vi "ChooseDualXDCRSettings.vi"(0 "Digitizer Settings in":T22={"Digitizer delay (us) "=0.0, "rf points per line"=0, "lines per plane"=0, "Samp Rate (Hz)"=0.0, "Additional dig delay (us)"=0.0, "Voltage Scale"=0.0, "Pre-Looks"=0, "Offset delay (us)"=0.0, "bits A/D"=0, "Avg Num"=0, "DigTimeOut"=0.0, "Rel Dig Delay"=0.0, "Dig Ch"=0, "LeCroyCluster"={"LeCroy Channels"=[], "LC read pt offset"=0.0, "Sweep Avg"=FALSE}, "Main Digitizer"=enum."Acqiris Digitizer", "Dig Config"=enum."Single channel", "Digitizer ID Cluster"={"Acqiris/Alazar/SP ID"=[], "NI Instr Handles"=[], "LeCroy VISA"="", "GaGe Handle"={"Handle"=0, "Sample size"=0, "Resolution"=0, "Offset"=0, "Channels"=0, "Boards"=0}, "ATS Ref"="ATS9350", "Acqiris Address"=["PCI::INSTR0"], "ADQRef"=refnum, "adq_cu_ptr"=refnum}, "Trigger Settings"={"Trig Source"=0, "Trig Coupling"=0, "Trig Slope"=0, "Level (mV)"=0.0}, "Bulk Acq"=FALSE, "Bulk Start Indexes"=[], "Data Ref RF"=refnum, "NI ID/Channel"=[], "Total Dig CH"=1, "Xtra Ann Trig delay (us)"=10.0, "Fix Z Delay?"=FALSE, "One Way Transmission?"=FALSE, "Data Ref Log"=refnum} {"Trigger Settings"."Trig Slope" items=["Positive", "Negative"]; "Trigger Settings"."Level (mV)" format="%.2f"; "Trigger Settings"."Trig Coupling" items=["DC 1 MOhm", "AC 1 MOhm", "DC 50 Ohm", "AC 50 Ohm"]; "Trigger Settings"."Trig Source" items=["Chan 1", "External"]; "Rel Dig Delay" format="%.2f"; "DigTimeOut" format="%.2f"; "Avg Num" min=1; "Offset delay (us)" format="%.2f"; "Additional dig delay (us)" format="%.2f"; "Digitizer delay (us)" format="%.2f"}, 1 "Switch T/R":u32=1, 2 "Set All UTEX?":bool=TRUE, 3 "Pulser":T1, 5 "Motion Settings in":T26={"No Motion?"=FALSE, "Motion System"=enum."MM3000", "Motion Bd ID"=0, "Motion Profile"="SMAC1", "# Axis"=0, "Reverse Z axis?"=FALSE, "SMAC Axis"=0, "scan pair"=enum."y-(x) scan", "RT fps"=0.0, "Steps per mm"=[], "Motor Parameters"={"velocity ct/s"=[], "accel ct/s^2"=[]}, "One Way Scan"=FALSE, "Reverse One Way Scan"=FALSE, "Global Position (mm)"=[], "Plane"=0, "Distance between\nscan lines (um)"=0.0, "Distance between\nscan planes (um)"=0.0, "number of scan planes"=0, "Total steps in line"=0, "Xtra plane\ndistance  (um)"=0, "Xtra planes "=0, "Add Axis"=FALSE, "overshoot cts"=0, "BKPT Shift"=0, "Scan Start Time (ms)"=0, "ESP VISA"="", "3rd Axis"=1, "GL Ref Out"=refnum, "Galil Address"=""} {"3rd Axis" items=["x", "y", "z", "w"]; "Xtra planes" min=1; "Xtra plane\ndistance  (um)" min=0; "Distance between\nscan planes (um)" format="%.2f"; "Distance between\nscan lines (um)" format="%.2f"; "SMAC Axis" items=["None"=0, "Axis 1"=1, "Axis 2"=2, "Axis 3"=3, "Axis 4"=4, "Axis 5"=5, "Axis 6"=6, "Axis 7"=7, "Axis 8"=8, "Vector Space 1"=17, "Vector Space 2"=18, "Vector Space 3"=19, "Vector Space 4"=20]; "Motion Bd ID" min=1 max=32 step=1}, 7 "Dual XDCR Settings":T2 {"XDCR Settings"."UT340 Controls"."Low Pass Filter (MHz)" min=-6 max=60 step=1; "XDCR Settings"."UT340 Controls"."High Pass Filter (MHz)" min=1 max=20 step=1; "XDCR Settings"."UT340 Controls"."Rep Rate (Hz)" min=20 step=1; "XDCR Settings"."UT340 Controls"."Pulse Width (ns)" min=100.0 max=250.0 step=2.0; "XDCR Settings"."UT340 Controls"."Voltage" min=100 max=250 step=2; "XDCR Settings"."UT340 Controls"."PC Gain (dB)" min=2 max=72; "XDCR Settings"."UT340 Controls"."PE Gain (dB)" min=-6 max=60 step=1; "XDCR Settings"."JSR Complete"."JSR Trigger Settings"."PRF (Hz)" items=["100 Hz"=0.1, "200 Hz"=0.2, "400 Hz"=0.4, "600 Hz"=0.6, "800 Hz"=0.8, "1000 Hz"=1.0, "1250 Hz"=1.25, "1500 Hz"=1.5, "1750 Hz"=1.75, "2000 Hz"=2.0, "2500 Hz"=2.5, "3000 Hz"=3.0, "3500 Hz"=3.5, "4000 Hz"=4.0, "4500 Hz"=4.5, "5000 Hz"=5.0]; "XDCR Settings"."JSR Complete"."JSR Trigger Settings"."Trigger Source" items=["Internal", "External"]; "XDCR Settings"."JSR Complete"."JSR Trigger Settings"."External Trigger Limit" items=["No Limit", "5 kHz"]; "XDCR Settings"."JSR Complete"."JSR Receive Settings"."Gain (dB)" min=-13 max=66 step=1; "XDCR Settings"."JSR Complete"."JSR Receive Settings"."Low Pass Filter" items=["5 MHz"=5, "10 MHz"=10, "15 MHz"=15, "22.5 MHz"=22, "35 MHz"=35, "50 MHz"=50]; "XDCR Settings"."JSR Complete"."JSR Receive Settings"."High Pass Filter" items=["DC"=0, "1 MHz"=1000, "2.5 MHz"=2500, "5 MHz"=5000, "7.5 MHz"=7500, "12.5 MHz"=12500]; "XDCR Settings"."JSR Complete"."JSR Receive Settings"."Receiver Mode" items=["Echo", "Through"]; "XDCR Settings"."JSR Complete"."JSR Pulse Settings"."Pulser Voltage (V)" items=["100"=100, "125"=125, "150"=150, "175"=175, "200"=200, "225"=225, "250"=250, "275"=275, "300"=300, "325"=325, "350"=350, "375"=375, "400"=400, "425"=425, "450"=450, "475"=475]; "XDCR Settings"."JSR Complete"."JSR Pulse Settings"."Pulser Impedance" items=["High z", "Low z"]; "XDCR Settings"."JSR Complete"."JSR Pulse Settings"."Pulse Energy Level" items=["0 (Minimum)", "1", "2", "3 (Maximum)"]; "XDCR Settings"."JSR Complete"."JSR Pulse Settings"."Damping" items=["331 Ohms"=331, "198 Ohms"=198, "142 Ohms"=142, "110 Ohms"=110, "92 Ohms"=92, "77 Ohms"=77, "67 Ohms"=67, "59 Ohms"=59, "52 Ohms"=52, "47 Ohms"=47, "43 Ohms"=43, "39 Ohms"=39, "37 Ohms"=37, "34 Ohms"=34, "32 Ohms"=32, "30 Ohms"=30]; "XDCR Settings"."Panametrics Settings"."FINE ATTENUATION" items=["00.0", "00.5", "01.0", "01.5", "02.0", "02.5", "03.0", "03.5", "04.0", "04.5", "05.0", "05.5", "06.0", "06.5", "07.0", "07.5", "08.0", "08.5", "09.0", "09.5", "10.0", "10.5", "11.0", "11.5", "12.0", "12.5", "13.0", "13.5", "14.0", "14.5", "15.0", "15.5"]; "XDCR Settings"."Panametrics Settings"."COARSE ATTENUATION" items=["00.0", "10.0", "20.0", "30.0", "40.0", "50.0"]; "XDCR Settings"."Panametrics Settings"."GAIN (db)" items=["26.0", "40.0", "54.0"]; "XDCR Settings"."Panametrics Settings"."PRF (KHz)" items=["XREMT", "EXBNC", "0.200", "0.500", "1.000", "2.000", "5.000", "10.00", "20.00"]; "XDCR Settings"."Panametrics Settings"."MODE" items=["P/ E", "THRU", "RPP", "EXT_PLSR"]; "XDCR Settings"."Panametrics Settings"."LP FILT (MHz)" items=["20", "50", "100", "200"]; "XDCR Settings"."Panametrics Settings"."HP FILT (KHz)" items=["1", "1000", "3000", "10000"]; "XDCR Settings"."Panametrics Settings"."DAMPING (Ohm)" items=["7", "10", "16", "20", "26", "30", "40", "50"]; "XDCR Settings"."Panametrics Settings"."ENERGY (uJ)" items=["1", "2", "4", "8", "16", "32"]; "XDCR Settings"."Daxsonics Settings"."Freq (MHz)" items=["4"=4, "5"=5, "6"=6, "8"=8, "10"=10, "12"=12, "14"=14, "15"=15, "16"=16, "17"=17, "18"=18, "20"=20, "25"=25, "30"=30, "35"=35, "40"=40, "45"=45, "50"=50]; "XDCR Settings"."Daxsonics Settings"."Voltage (V)" items=["0"=0, "5"=5, "10"=10, "15"=15, "20"=20, "25"=25, "30"=30, "35"=35, "40"=40, "45"=45, "50"=50, "55"=55, "60"=60, "65"=65, "70"=70, "75"=75, "80"=80, "85"=85, "90"=90, "95"=95, "100"=100, "110"=110, "120"=120, "130"=130, "140"=140, "150"=150, "160"=160, "170"=170, "180"=180, "190"=190]; "XDCR Settings"."Daxsonics Settings"."Gain (dB)" items=["22"=22, "25"=25, "28"=28, "31"=31, "34"=34, "37"=37, "40"=40, "43"=43, "46"=46, "49"=49, "52"=52, "55"=55, "58"=58, "61"=61, "64"=64, "67"=67]; "XDCR Settings"."Digitizer Settings"."Additional dig delay (ms)" format="%.2f"; "XDCR Settings"."Digitizer Settings"."Time scale per Div" items=["100 ns"=0.1, "200 ns"=0.2, "500 ns"=0.5, "1 micros"=1.0, "2 micros"=2.0, "5 micros"=5.0, "10 micros"=10.0, "20 micros"=20.0, "50 micros"=50.0, "100 micros"=100.0, "200 micros"=200.0, "500 micros"=500.0, "1 ms"=1000.0, "2 ms"=2000.0, "5 ms"=5000.0, "10 ms"=10000.0, "20 ms"=20000.0, "50 ms"=50000.0, "100 ms"=100000.0, "200 ms"=200000.0]; "XDCR Settings"."Digitizer Settings"."RF data Sampling"."rf points per line" min=1; "XDCR Settings"."Digitizer Settings"."RF data Sampling"."Ref Delay (ms)" format="%.2f"}, 8 "Setup Time\nParameters (F)":bool, 9 "Allow USB R/Ws?":bool=TRUE, 10 "JSR Simple":refnum<vi>, 11 "JSR Complete":refnum<vi>, 12 "Time scale per Div Ref":refnum<vi>, 13 "RF data Sampling Ref":refnum<vi>, 14 "Filter Parameters Ref":refnum<vi>, 15 "Daxsonics Settings Ref":refnum<vi>, 16 "Panametrics Simple Ref":refnum<vi>, 17 "Panametrics Settings Ref":refnum<vi>, 18 "UT340 Simple Ref":refnum<vi>, 19 "UT340 Ref":refnum<vi>) -> (20 "Digitizer Settings":T22={"Digitizer delay (us) "=0.0, "rf points per line"=0, "lines per plane"=0, "Samp Rate (Hz)"=0.0, "Additional dig delay (us)"=0.0, "Voltage Scale"=0.0, "Pre-Looks"=0, "Offset delay (us)"=0.0, "bits A/D"=0, "Avg Num"=0, "DigTimeOut"=0.0, "Rel Dig Delay"=0.0, "Dig Ch"=0, "LeCroyCluster"={"LeCroy Channels"=[], "LC read pt offset"=0.0, "Sweep Avg"=FALSE}, "Main Digitizer"=enum."Acqiris Digitizer", "Dig Config"=enum."Single channel", "Digitizer ID Cluster"={"Acqiris/Alazar/SP ID"=[], "NI Instr Handles"=[], "LeCroy VISA"="", "GaGe Handle"={"Handle"=0, "Sample size"=0, "Resolution"=0, "Offset"=0, "Channels"=0, "Boards"=0}, "ATS Ref"="ATS9350", "Acqiris Address"=["PCI::INSTR0"], "ADQRef"=refnum, "adq_cu_ptr"=refnum}, "Trigger Settings"={"Trig Source"=0, "Trig Coupling"=0, "Trig Slope"=0, "Level (mV)"=0.0}, "Bulk Acq"=FALSE, "Bulk Start Indexes"=[], "Data Ref RF"=refnum, "NI ID/Channel"=[], "Total Dig CH"=1, "Xtra Ann Trig delay (us)"=10.0, "Fix Z Delay?"=FALSE, "One Way Transmission?"=FALSE, "Data Ref Log"=refnum} {"Trigger Settings"."Trig Slope" items=["Positive", "Negative"]; "Trigger Settings"."Level (mV)" format="%.2f"; "Trigger Settings"."Trig Coupling" items=["DC 1 MOhm", "AC 1 MOhm", "DC 50 Ohm", "AC 50 Ohm"]; "Trigger Settings"."Trig Source" items=["Chan 1", "External"]; "Rel Dig Delay" format="%.2f"; "DigTimeOut" format="%.2f"; "Avg Num" min=1; "Offset delay (us)" format="%.2f"; "Additional dig delay (us)" format="%.2f"; "Digitizer delay (us)" format="%.2f"}, 21 "Change Polarity":i32, 25 "Motion Settings":T26={"No Motion?"=FALSE, "Motion System"=enum."MM3000", "Motion Bd ID"=0, "Motion Profile"="SMAC1", "# Axis"=0, "Reverse Z axis?"=FALSE, "SMAC Axis"=0, "scan pair"=enum."y-(x) scan", "RT fps"=0.0, "Steps per mm"=[], "Motor Parameters"={"velocity ct/s"=[], "accel ct/s^2"=[]}, "One Way Scan"=FALSE, "Reverse One Way Scan"=FALSE, "Global Position (mm)"=[], "Plane"=0, "Distance between\nscan lines (um)"=0.0, "Distance between\nscan planes (um)"=0.0, "number of scan planes"=0, "Total steps in line"=0, "Xtra plane\ndistance  (um)"=0, "Xtra planes "=0, "Add Axis"=FALSE, "overshoot cts"=0, "BKPT Shift"=0, "Scan Start Time (ms)"=0, "ESP VISA"="", "3rd Axis"=1, "GL Ref Out"=refnum, "Galil Address"=""} {"3rd Axis" items=["x", "y", "z", "w"]; "Xtra planes" min=1; "Xtra plane\ndistance  (um)" min=0; "Distance between\nscan planes (um)" format="%.2f"; "Distance between\nscan lines (um)" format="%.2f"; "SMAC Axis" items=["None"=0, "Axis 1"=1, "Axis 2"=2, "Axis 3"=3, "Axis 4"=4, "Axis 5"=5, "Axis 6"=6, "Axis 7"=7, "Axis 8"=8, "Vector Space 1"=17, "Vector Space 2"=18, "Vector Space 3"=19, "Vector Space 4"=20]; "Motion Bd ID" min=1 max=32 step=1})   [LabVIEW 2022 SP3]
uses:
  Motion Controllers/NI_controller/-NI_MotionRoutines/MotionParameters.ctl
  Motion Controllers/NI_controller/-NI_MotionRoutines/MotionSys.ctl
  Motion Controllers/-MotionRoutines/ScanAxis.ctl
  Motion Controllers/-MotionRoutines/3rdAxis.ctl
  Digitizers/-DigitizerRoutines/DigitizerSettings.ctl
  Digitizers/-DigitizerRoutines/Digitizer.ctl
  Digitizers/-DigitizerRoutines/DigConfig.ctl
  Digitizers/-DigitizerRoutines/DigitizerID.ctl
  C:/Windows/System32/ADQAPI_dotNet_helper.dll
  Windows/System32/ADQAPI_dotNet_helper.dll
  Dual XDCR Complete Settings.ctl
  XDCRSettings.ctl
  Pulsers/Daxsonics/-DaxSubroutines/Dax_Control_Cluster.ctl
  Pulsers/Panametrics/Pana5900.ctl
  Pulsers/JSR/Controls/JSR Complete.ctl
  Pulsers/JSR/Controls/JSR Pulse.ctl
  Pulsers/JSR/Controls/Damping.ctl
  Pulsers/JSR/Controls/Energy.ctl
  Pulsers/JSR/Controls/Z.ctl
  Pulsers/JSR/Controls/Volt.ctl
  Pulsers/JSR/Controls/JSR Recieve.ctl
  Pulsers/JSR/Controls/Mode.ctl
  Pulsers/JSR/Controls/HPF.ctl
  Pulsers/JSR/Controls/LPF.ctl
  Pulsers/JSR/Controls/Gain.ctl
  Pulsers/JSR/Controls/JSR Trigger.ctl
  Pulsers/JSR/Controls/Trig Limit.ctl
  Pulsers/JSR/Controls/Trig Source.ctl
  Pulsers/JSR/Controls/PRF.ctl
  Pulsers/UTEX/Controls/UTEX Controls.ctl
  Pulsers/pulser.ctl
  Pulsers/JSR/Controls/JSR Simple.ctl
  Pulsers/UTEX/Controls/UTEX Controls Simple.ctl
  Pulsers/PulserGlobals.vi
panel:
  # "1-D and 2-D B scan settings"
  # "1-D and 2-D B scan settings"
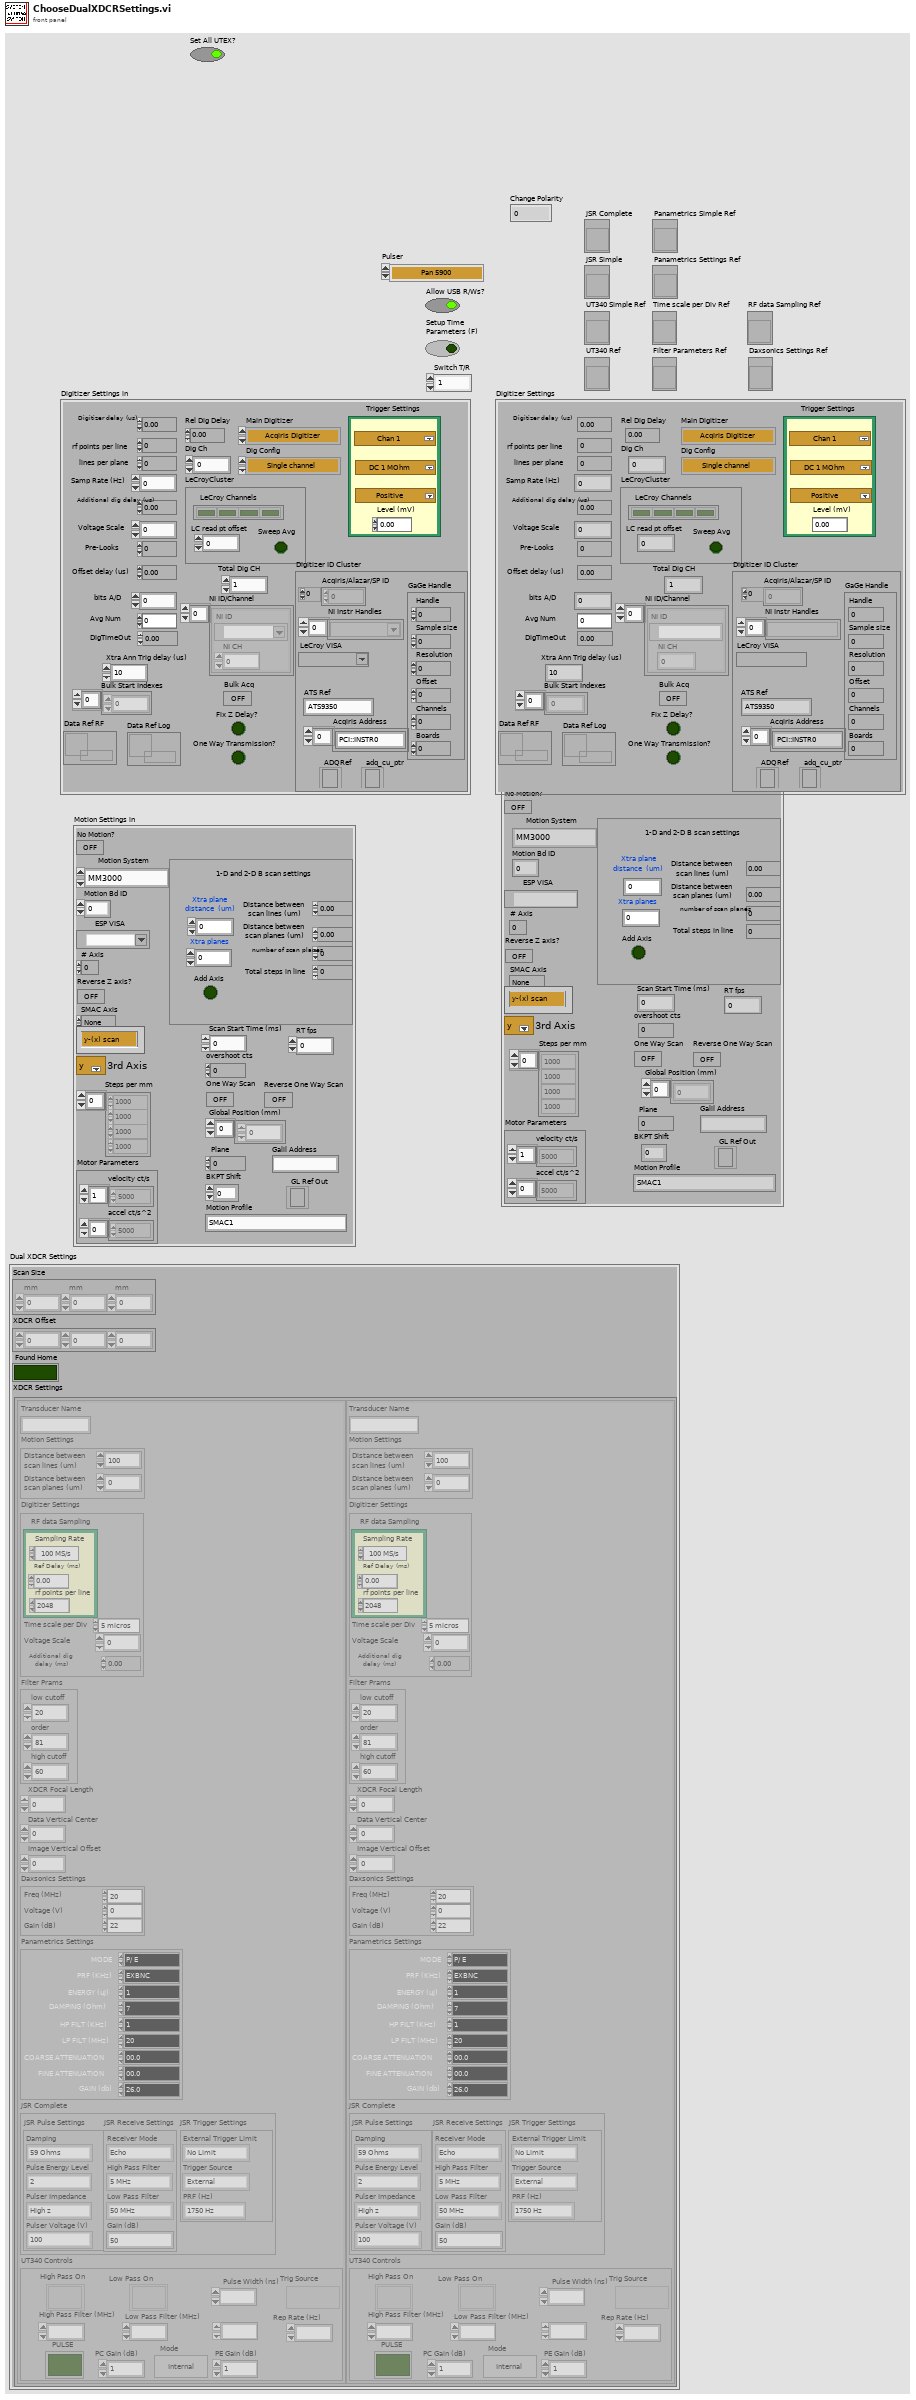
[diagram p1: front panel]
types:
  T1 = typedef "pulser.ctl" = enum16{"Pan 5900", "Daxsonics", "Agilent 33xxx", "UTEX", "JSR", "WMC Mono-Cycle", "No Pulser", "NYU AVTECH", "Tabor W1281A", "Pan 5800", "Unlisted", "Tabor WX2182B"}
  T2 = typedef "Dual XDCR Complete Settings.ctl" = cluster{"Scan Size":dbl[], "XDCR Offset":dbl[], "Found Home":bool, "XDCR Settings":T3[]}
  T3 = typedef "XDCRSettings.ctl" = cluster{"Transducer Name":string, "Motion Settings":cluster{"Distance between\nscan lines (um)":sgl, "Distance between\nscan planes (um)":sgl}, "Digitizer Settings":cluster{"RF data Sampling":cluster{"Sampling Rate":dbl, "Ref Delay (ms)":dbl, "rf points per line":i32}, "Time scale per Div":dbl, "Voltage Scale":dbl, "Additional dig delay (ms)":dbl}, "Filter Prams":cluster{"low cutoff":i32, "order":i32, "high cutoff":i32}, "XDCR Focal Length":dbl, "Data Vertical Center":dbl, "Image Vertical Offset":dbl, "Daxsonics Settings":T4, "Panametrics Settings":T5, "JSR Complete":T6, "UT340 Controls":T21}
  T4 = typedef "Dax_Control_Cluster.ctl" = cluster{"Freq (MHz) ":u16, "Voltage (V)":u16, "Gain (dB)":u16}
  T5 = typedef "Pana5900.ctl" = cluster{"ENERGY (uJ)":u16, "DAMPING (Ohm)":u16, "HP FILT (KHz) ":u16, "LP FILT (MHz)":u16, "MODE":u16, "PRF (KHz)":u16, "GAIN (db)":u16, "COARSE ATTENUATION":u16, "FINE ATTENUATION":u16}
  T6 = typedef "JSR Complete.ctl" = cluster{"JSR Pulse Settings":T7, "JSR Receive Settings":T12, "JSR Trigger Settings":T17}
  T7 = typedef "JSR Pulse.ctl" = cluster{"Damping":T8, "Pulse Energy Level":T9, "Pulser Impedance":T10, "Pulser Voltage (V)":T11}
  T8 = typedef "Damping.ctl" = i16
  T9 = typedef "Energy.ctl" = u16
  T10 = typedef "Z.ctl" = u16
  T11 = typedef "Volt.ctl" = i16
  T12 = typedef "JSR Recieve.ctl" = cluster{"Receiver Mode":T13, "High Pass Filter":T14, "Low Pass Filter":T15, "Gain (dB)":T16}
  T13 = typedef "Mode.ctl" = i8
  T14 = typedef "HPF.ctl" = u16
  T15 = typedef "LPF.ctl" = u16
  T16 = typedef "Gain.ctl" = i8
  T17 = typedef "JSR Trigger.ctl" = cluster{"External Trigger Limit":T18, "Trigger Source":T19, "PRF (Hz)":T20}
  T18 = typedef "Trig Limit.ctl" = i8
  T19 = typedef "Trig Source.ctl" = i8
  T20 = typedef "PRF.ctl" = dbl
  T21 = typedef "UTEX Controls.ctl" = cluster{"High Pass On":bool, "High Pass Filter (MHz)":i16, "Low Pass On":bool, "Low Pass Filter (MHz)":i16, "PE Gain (dB)":i16, "Voltage":i16, "Pulse Width (ns)":dbl, "Mode":bool, "PC Gain (dB)":i16, "Trig Source":bool, "Rep Rate (Hz)":i16, "PULSE":bool}
  T22 = typedef "DigitizerSettings.ctl" = cluster{"Digitizer delay (us) ":dbl, "rf points per line":i32, "lines per plane":i32, "Samp Rate (Hz)":dbl, "Additional dig delay (us)":dbl, "Voltage Scale":dbl, "Pre-Looks":i32, "Offset delay (us)":dbl, "bits A/D":i8, "Avg Num":i32, "DigTimeOut":sgl, "Rel Dig Delay":sgl, "Dig Ch":i32, "LeCroyCluster":cluster{"LeCroy Channels":bool[], "LC read pt offset":dbl, "Sweep Avg":bool}, "Main Digitizer":T23, "Dig Config":T24, "Digitizer ID Cluster":T25, "Trigger Settings":cluster{"Trig Source":u16, "Trig Coupling":u16, "Trig Slope":u16, "Level (mV)":dbl}, "Bulk Acq":bool, "Bulk Start Indexes":i32[], "Data Ref RF":refnum<data-value>, "NI ID/Channel":cluster{"NI ID":refnum<k15>, "NI CH":i32}[], "Total Dig CH":i32, "Xtra Ann Trig delay (us)":dbl, "Fix Z Delay?":bool, "One Way Transmission?":bool, "Data Ref Log":refnum<data-value>}
  T23 = typedef "Digitizer.ctl" = enum16{"Acqiris Digitizer", "NI Digitizer", "LeCroy", "GaGe", "AlazarTech", "No Digitizer", "Teledyne"}
  T24 = typedef "DigConfig.ctl" = enum16{"Single channel", "2 Chans w/ 2 Acqiris", "2 Chans w/ 1 Acqiris", "5-CH Pulser New", "5-CH pulser w/ ann array", "5-pass style ann array", "Empty"}
  T25 = typedef "DigitizerID.ctl" = cluster{"Acqiris/Alazar/SP ID":u32[], "NI Instr Handles":refnum<k15>[], "LeCroy VISA":refnum<visa-resource-name>, "GaGe Handle":cluster{"Handle":u32, "Sample size":u32, "Resolution":i32, "Offset":i32, "Channels":u32, "Boards":u32}, "ATS Ref":string, "Acqiris Address":string[], "ADQRef":refnum<k24>, "adq_cu_ptr":refnum<k24>}
  T26 = typedef "MotionParameters.ctl" = cluster{"No Motion?":bool, "Motion System":T27, "Motion Bd ID":u8, "Motion Profile":string, "# Axis":i8, "Reverse Z axis?":bool, "SMAC Axis":u16, "scan pair":T28, "RT fps":sgl, "Steps per mm":i32[], "Motor Parameters":cluster{"velocity ct/s":dbl[], "accel ct/s^2":dbl[]}, "One Way Scan":bool, "Reverse One Way Scan":bool, "Global Position (mm)":dbl[], "Plane":i32, "Distance between\nscan lines (um)":sgl, "Distance between\nscan planes (um)":sgl, "number of scan planes":i32, "Total steps in line":i32, "Xtra plane\ndistance  (um)":i32, "Xtra planes ":i32, "Add Axis":bool, "overshoot cts":i32, "BKPT Shift":i32, "Scan Start Time (ms)":u32, "ESP VISA":refnum<visa-resource-name>, "3rd Axis":T29, "GL Ref Out":refnum<k7>, "Galil Address":string}
  T27 = typedef "MotionSys.ctl" = enum16{"MM3000", "NI 735x", "Newport ESP", "No Motion Card", "Galil"}
  T28 = typedef "ScanAxis.ctl" = enum16{"y-(x) scan", "x-(y) scan", "z-(x) scan", "z-(y) scan", "y-(z) scan", "x-(z) scan", "w-(x) scan", "w-(y) scan", "w-(z) scan", "x-(w) scan", "y-(w) scan", "z-(w) scan"}
  T29 = typedef "3rdAxis.ctl" = u16
  T30 = cluster{"ENERGY (uJ)":u16, "COARSE ATTENUATION":u16, "FINE ATTENUATION":u16}
  T31 = cluster{"High Pass On":bool, "High Pass Filter (MHz)":bool, "Low Pass On":bool, "Low Pass Filter (MHz)":bool, "PE Gain (dB)":bool, "Voltage":bool, "Pulse Width (ns)":bool, "Mode":bool, "PC Gain (dB)":bool, "Trig Source":bool, "Rep Rate (Hz)":bool, "PULSE":bool}
  T32 = cluster{"RF data Sampling":cluster{"Sampling Rate":dbl, "Ref Delay (ms)":dbl, "rf points per line":i32}, "Time scale per Div":dbl, "Voltage Scale":dbl, "Additional dig delay (ms)":dbl}
  T33 = cluster{"Distance between\nscan lines (um)":sgl, "Distance between\nscan planes (um)":sgl}
  T34 = cluster{"low cutoff":i32, "order":i32, "high cutoff":i32}
  T35 = typedef "JSR Simple.ctl" = cluster{"Pulse Energy Level":T9, "Gain (dB)":T16, "Pulser Voltage (V)":T11}
  T36 = typedef "UTEX Controls Simple.ctl" = cluster{"PE Gain (dB)":i16, "Voltage":i16}
  T37 = cluster{"Sampling Rate":dbl, "Ref Delay (ms)":dbl, "rf points per line":i32}
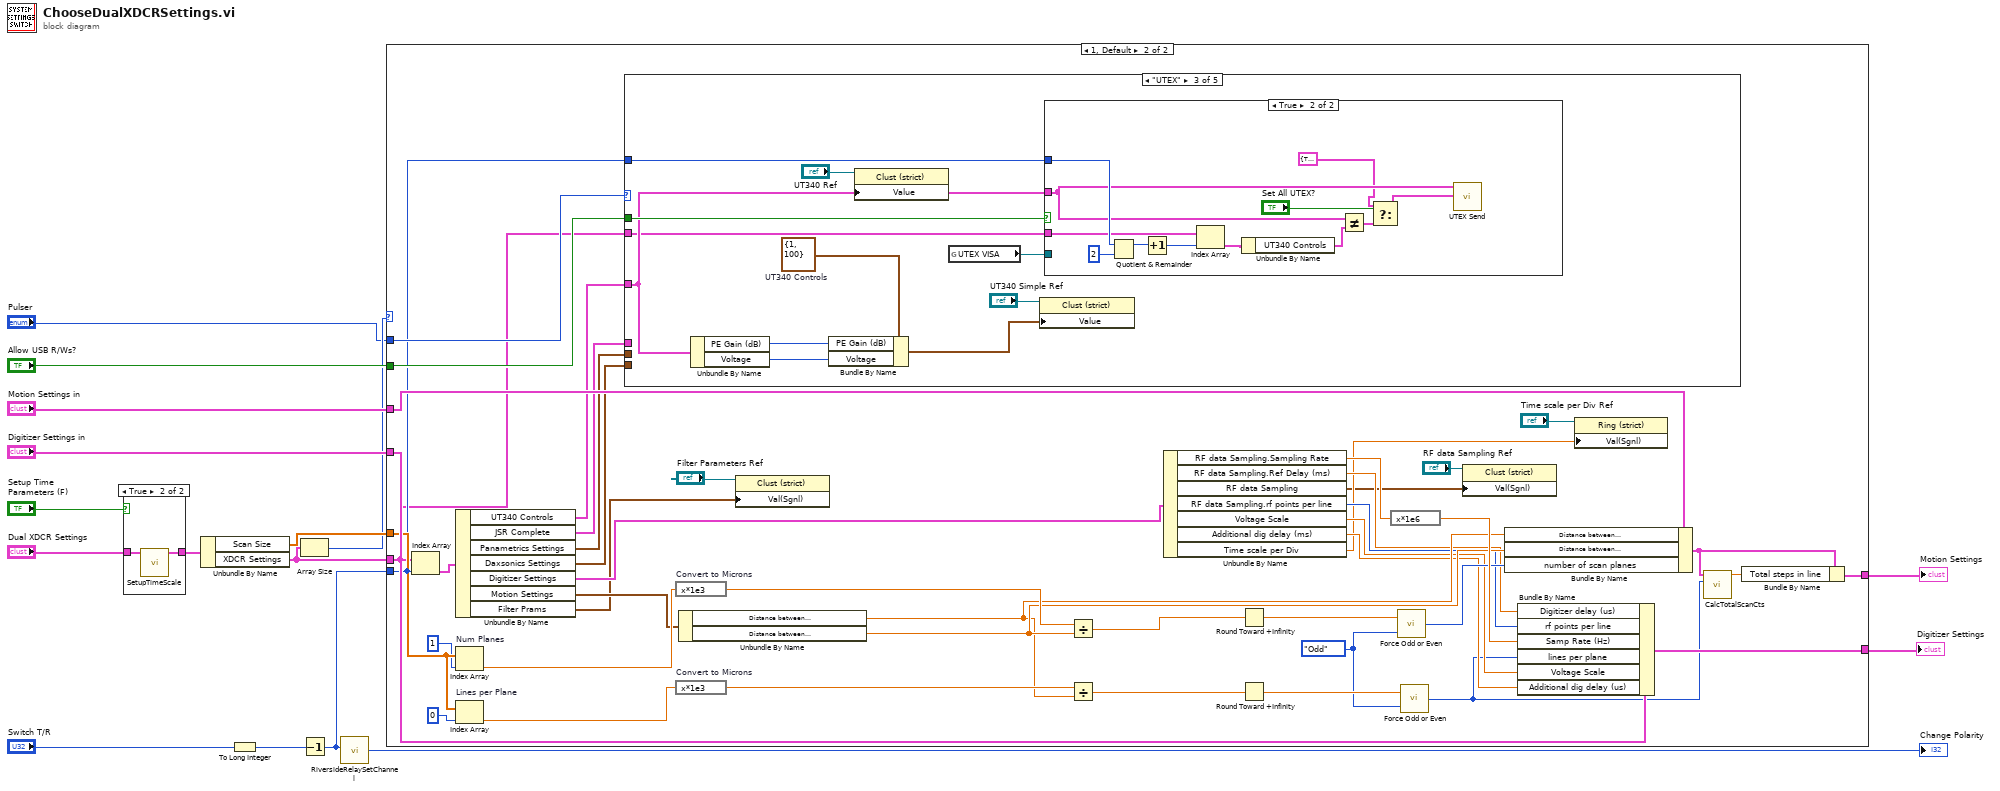
[diagram p0: block diagram]
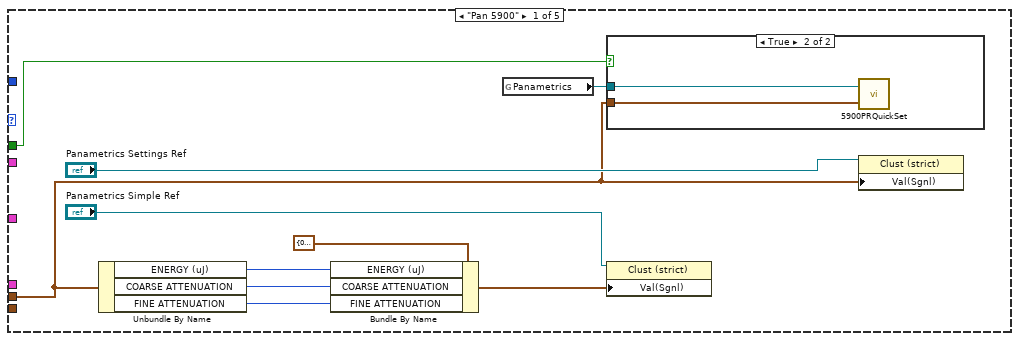
[diagram p3: hidden frame]
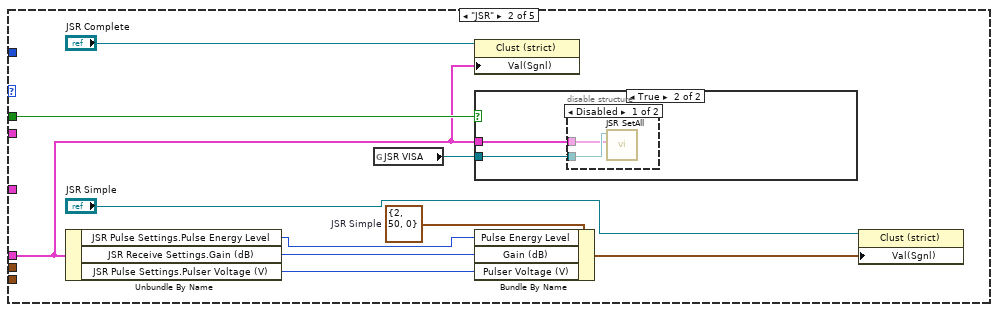
[diagram p5: hidden frame]
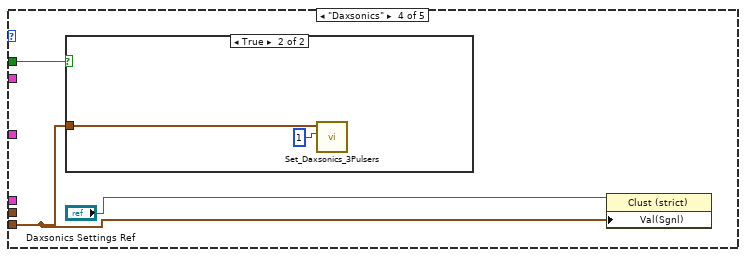
[diagram p9: hidden frame]
diagram:
  n1 = case shown="True" "Setup Time\nParameters (F)" {
    tunnel: "Dual XDCR Settings" -> [w17 w19]
    tunnel: [w17 w18] -> w10
    frame False {
    }
    frame True {
      n2 = call "SetupTimeScale.vi"("Dual XDCR Settings in"=w19) -> ("Dual XDCR Settings out"=w18:T2)  [unwired: 10 in]
    }
  }
  n3 = Unbundle By Name(w10) -> ("Scan Size"=w8:dbl[], "XDCR Settings"=w3:T3[])
  n4 = To Long Integer(number="Switch T/R") -> (32bit integer=w13:i32)
  n5 = Array Size(array=w3) -> (size(s)=w2:i32)
  n6 = Decrement(x=w13) -> (x-1=w5:i32)
  n7 = call "RiversideRelaySetChannel.vi"("Transducer"=w5) -> ("Change Polarity"=→"Change Polarity":i32)  [unwired: 4 in, 2 out]
  n8 = case shown="1, Default" w2 {
    tunnel: [w20 w66] -> w16
    tunnel: "Digitizer Settings in" -> [w20 w65]
    tunnel: "Motion Settings in" -> [w21 w64]
    tunnel: w8 -> [_ w63]
    tunnel: [w21 w62] -> w7
    tunnel: w3 -> [_ w22]
    tunnel: "Allow USB R/Ws?" -> [_ w61]
    tunnel: w5 -> [_ w23]
    tunnel: "Pulser" -> [_ w27]
    frame 0 {
    }
    frame 1, Default {
      w50 = enum16{"Odd", "Even"}."Odd" ("Parity")
      n9 = Index Array(array=w22, index=w23) -> (element=w37:T3)
      n10 = Unbundle By Name(w37) -> ("UT340 Controls"=w24:T21, "JSR Complete"=w25:T6, "Panametrics Settings"=w26:T5, "Daxsonics Settings"=w28:T4, "Digitizer Settings"=w36:T32, "Motion Settings"=w35:T33, "Filter Prams"=w31:T34)
      n11 = Index Array "Num Planes"(array=w63, index=1) -> (element=w43:dbl)
      n12 = Index Array "Lines per Plane"(array=w63, index=0) -> (element=w46:dbl)
      n13 = case shown="\"UTEX\"" w27 {
        tunnel: w61 -> [w67 w87 w102 w118 _]
        tunnel: w28 -> [_ _ _ w117 _]
        tunnel: w26 -> [w71 _ _ _ _]
        tunnel: w25 -> [_ w82 _ _ _]
        tunnel: w24 -> [_ _ w95 _ _]
        tunnel: w23 -> [_ _ w94 _ _]
        tunnel: w22 -> [_ _ w93 _ _]
        frame "Pan 5900" {
          n14 = Unbundle By Name(w71) -> ("ENERGY (uJ)"=w70:u16, "COARSE ATTENUATION"=w69:u16, "FINE ATTENUATION"=w68:u16)
          n15 = Bundle By Name(cluster=T30 {"ENERGY (uJ)"=0, "COARSE ATTENUATION"=0, "FINE ATTENUATION"=0} ("Panametrics Settings Simple"), "ENERGY (uJ)"=w70, "COARSE ATTENUATION"=w69, "FINE ATTENUATION"=w68) -> (w74:T30)
          n16 = global read "PulserGlobals.vi" "Panametrics"() -> (w76:refnum<visa-resource-name>)
          n17 = case shown="True" w67 {
            tunnel: w76 -> [_ w78]
            tunnel: w71 -> [_ w77]
            frame False {
            }
            frame True {
              n18 = call "5900PRQuickSet.vi"("VISA resource name"=w78, "Panametrics Settings"=w77) -> ()  [unwired: 2 in, 1 out]
            }
          }
          n19 = property class="Clust (strict)"(reference="Panametrics Simple Ref", "Val(Sgnl)"=w74) -> ()  [unwired: 1 in, 2 out]
          n20 = property class="Clust (strict)"(reference="Panametrics Settings Ref", "Val(Sgnl)"=w71) -> ()  [unwired: 1 in, 2 out]
        }
        frame "JSR" {
          w83 = T35 {"Pulse Energy Level"=2, "Gain (dB)"=50, "Pulser Voltage (V)"=0}  # JSR Simple
          n21 = Unbundle By Name(w82) -> ("JSR Pulse Settings.Pulse Energy Level"=w81:T9, "JSR Receive Settings.Gain (dB)"=w79:T16, "JSR Pulse Settings.Pulser Voltage (V)"=w80:T11)
          n22 = global read "PulserGlobals.vi" "JSR VISA"() -> (w88:refnum<visa-resource-name>)
          n23 = property class="Clust (strict)"(reference="JSR Complete", "Val(Sgnl)"=w82) -> ()  [unwired: 1 in, 2 out]
          n24 = case shown="True" w87 {
            tunnel: w88 -> [_ w90]
            tunnel: w82 -> [_ w89]
            frame False {
            }
            frame True {
              n25 = disable-structure shown="Disabled" {
                disable-tunnel: w90 -> [w92 _]
                disable-tunnel: w89 -> [w91 _]
                frame Disabled {
                  n26 = call "JSR SetAll.vi"("JSR Complete"=w91, "JSR VISA"=w92) -> ()  [unwired: 8 in, 2 out]
                }
                frame Enabled {
                }
              }
            }
          }
          n27 = Bundle By Name(cluster=w83, "Pulse Energy Level"=w81, "Gain (dB)"=w79, "Pulser Voltage (V)"=w80) -> (w84:T35)
          n28 = property class="Clust (strict)"(reference="JSR Simple", "Val(Sgnl)"=w84) -> ()  [unwired: 1 in, 2 out]
        }
        frame "UTEX" {
          w101 = T36 {"PE Gain (dB)"=1, "Voltage"=100}  # UT340 Controls
          n29 = Unbundle By Name(w95) -> ("PE Gain (dB)"=w97:i16, "Voltage"=w96:i16)
          n30 = Bundle By Name(cluster=w101, "PE Gain (dB)"=w97, "Voltage"=w96) -> (w99:T36)
          n31 = property class="Clust (strict)"(reference="UT340 Ref", "Value"=w95) -> ()  [unwired: 1 in, 2 out]
          n32 = global read "PulserGlobals.vi" "UTEX VISA"() -> (w103:refnum<visa-resource-name>)
          n33 = property class="Clust (strict)"(reference="UT340 Simple Ref", "Value"=w99) -> ()  [unwired: 1 in, 2 out]
          n34 = case shown="True" w102 {
            tunnel: w103 -> [_ _]
            tunnel: w95 -> [_ w108]
            tunnel: w94 -> [_ w112]
            tunnel: w93 -> [_ w110]
            frame False {
            }
            frame True {
              n35 = Quotient & Remainder(x=w112, y=2) -> (x-y*floor(x/y)=w115:i32)  [unwired: 1 out]
              n36 = Increment(x=w115) -> (x+1=w114:i32)
              n37 = Index Array(array=w110, index=w114) -> (element=w111:T3)
              n38 = Unbundle By Name(w111) -> ("UT340 Controls"=w109:T21)
              n39 = Not Equal?(x=w108, y=w109) -> (x != y?=w107:T31)
              n40 = Select(t=T31 {"High Pass On"=TRUE, "High Pass Filter (MHz)"=TRUE, "Low Pass On"=TRUE, "Low Pass Filter (MHz)"=TRUE, "PE Gain (dB)"=TRUE, "Voltage"=TRUE, "Pulse Width (ns)"=TRUE, "Mode"=TRUE, "PC Gain (dB)"=TRUE, "Trig Source"=TRUE, "Rep Rate (Hz)"=TRUE, "PULSE"=TRUE}, s="Set All UTEX?", f=w107) -> (s? t:f=w106:T31)
              n41 = call "UTEX Send.vi"("Changed Values?"=w106, "UT340 Controls"=w108) -> ()  [unwired: 9 in, 1 out]
            }
          }
        }
        frame "Daxsonics" {
          n42 = case shown="True" w118 {
            tunnel: w117 -> [_ w120]
            frame False {
            }
            frame True {
              n43 = call "Set_Daxsonics_3Pulsers.vi"("Number of Channels"=1, "Daxsonics Settings"=w120) -> ()  [unwired: 8 in]
            }
          }
          n44 = property class="Clust (strict)"(reference="Daxsonics Settings Ref", "Val(Sgnl)"=w117) -> ()  [unwired: 1 in, 2 out]
        }
        frame Default {
        }
      }
      n45 = expression code="x*1e3" "Convert to Microns"(w43) -> (w59:dbl)
      n46 = expression code="x*1e3" "Convert to Microns"(w46) -> (w55:dbl)
      n47 = Unbundle By Name(w35) -> ("Distance between\nscan lines (um)"=w54:sgl, "Distance between\nscan planes (um)"=w58:sgl)
      n48 = property class="Clust (strict)"(reference="Filter Parameters Ref", "Val(Sgnl)"=w31) -> ()  [unwired: 1 in, 2 out]
      n49 = Divide(x=w59, y=w58) -> (x/y=w57:dbl)
      n50 = Divide(x=w55, y=w54) -> (x/y=w56:dbl)
      n51 = Unbundle By Name(w36) -> ("RF data Sampling.Sampling Rate"=w48:dbl, "RF data Sampling.Ref Delay (ms)"=w49:dbl, "RF data Sampling"=w29:T37, "RF data Sampling.rf points per line"=w47:i32, "Voltage Scale"=w42:dbl, "Additional dig delay (ms)"=w41:dbl, "Time scale per Div"=w34:dbl)
      n52 = Round Toward +Infinity(x=w57) -> (ceil(x): smallest int >= x=w52:dbl)
      n53 = Round Toward +Infinity(x=w56) -> (ceil(x): smallest int >= x=w53:dbl)
      n54 = expression code="x*1e6"(w48) -> (w60:dbl)
      n55 = call "Force Odd or Even.vi"("Parity (odd)"=w50, "input"=w52) -> ("output"=w51:i32)
      n56 = call "Force Odd or Even.vi"("Parity (odd)"=w50, "input"=w53) -> ("output"=w40:i32)
      n57 = property class="Clust (strict)"(reference="RF data Sampling Ref", "Val(Sgnl)"=w29) -> ()  [unwired: 1 in, 2 out]
      n58 = Bundle By Name(cluster=w64, "Distance between\nscan lines (um)"=w54, "Distance between\nscan planes (um)"=w58, "number of scan planes"=w51) -> (w39:T26)
      n59 = Bundle By Name(cluster=w65, "Digitizer delay (us)"=w49, "rf points per line"=w47, "Samp Rate (Hz)"=w60, "lines per plane"=w40, "Voltage Scale"=w42, "Additional dig delay (us)"=w41) -> (w66:T22)
      n60 = property class="Ring (strict)"(reference="Time scale per Div Ref", "Val(Sgnl)"=w34) -> ()  [unwired: 1 in, 2 out]
      n61 = call "CalcTotalScanCts.vi"("Number of scan lines"=w40, "Motion Settings In"=w39) -> ("Total Steps"=w38:dbl)  [unwired: 9 in]
      n62 = Bundle By Name(cluster=w39, "Total steps in line"=w38) -> (w62:T26)
    }
  }
  "Motion Settings" <- w7
  "Digitizer Settings" <- w16
